vi "ConcatTwoStrings.vi"(9 "String 2":string, 11 "String":string) -> (3 "String 3":string)   [LabVIEW 2012]
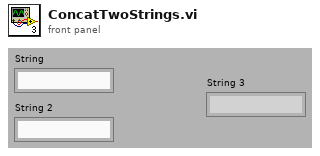
[diagram p1: front panel]
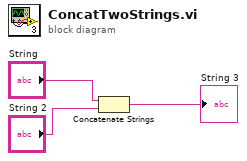
[diagram p0: block diagram]
diagram:
  n1 = Concatenate Strings("String", "String 2") -> (→"String 3":string)
